vi "Handle Lask Ack.vi"(8 "error in (no error)":errorcluster, 10 "Last Ack":refnum<class "Last Ack.lvclass">, 11 "cRIO-CO2 in":refnum<class "cRIO-CO2.lvclass">) -> (0 "error out":errorcluster, 3 "cRIO-CO2 out":refnum<class "cRIO-CO2.lvclass">)   [LabVIEW 2015, in "cRIO-Carbondioxide.lvlib" / "cRIO-CO2.lvlib" / "cRIO-CO2.lvclass"]
uses:
  cRIO-CO2.lvclass
  <vilib>/ActorFramework/LastAck/Last Ack.lvclass
  CO2 Actor/CO2 Actor.lvclass
  <vilib>/ActorFramework/LastAck/Last Ack.lvclass/Last Ack.ctl
  CO2 Actor/CO2 Actor.lvclass/CO2 Actor.ctl
  cRIO-CO2.lvclass/cRIO-CO2.ctl
  <vilib>/ActorFramework/Message Enqueuer/Message Enqueuer.lvclass/Message Enqueuer.ctl
  <vilib>/ActorFramework/Message Enqueuer/Enqueue.vi
  <vilib>/ActorFramework/Message Priority Queue/Priority Enqueue.vi
  <vilib>/ActorFramework/Stop Msg/Stop Msg.lvclass
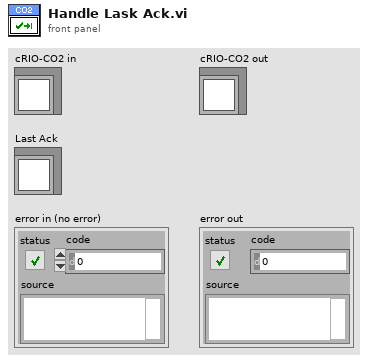
[diagram p1: front panel]
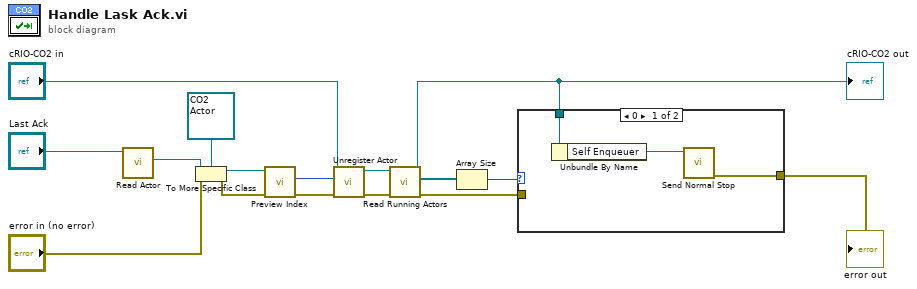
[diagram p0: block diagram]
diagram:
  n1 = call <vilib>:"Read Actor.vi"("Last Ack"="Last Ack") -> ("Actor"=w14:refnum<class "Actor.lvclass">)  [unwired: 10 in]
  n2 = To More Specific Class(target class=refnum<class "CO2 Actor.lvclass"> refnum ("CO2 Actor.lvclass"), reference=w14, error in="error in (no error)") -> (specific class reference=w12:refnum<class "CO2 Actor.lvclass">, error out=w13:errorcluster)
  n3 = call "Preview Index.vi"("error in (no error)"=w13, "CO2 Actor in"=w12) -> ("error out"=w11:errorcluster, "Index"=w9:i32)  [unwired: 7 in, 1 out]
  n4 = call "Unregister Actor.vi"("error in (no error)"=w11, "Index"=w9, "cRIO-CO2 in"="cRIO-CO2 in") -> ("error out"=w8:errorcluster, "cRIO-CO2 out"=w7:refnum<class "cRIO-CO2.lvclass">)  [unwired: 7 in]
  n5 = call "Read Running Actors.vi"("error in (no error)"=w8, "cRIO-CO2 in"=w7) -> ("error out"=w2:errorcluster, "Running Actors"=w6:refnum<class "CO2 Actor.lvclass">[], "cRIO-CO2 out"=w4:refnum<class "cRIO-CO2.lvclass">)  [unwired: 7 in]
  "cRIO-CO2 out" <- w4
  n6 = Array Size(array=w6) -> (size(s)=w5:i32)
  n7 = case shown="0" w5 {
    tunnel: w4 -> [w19 _]
    tunnel: [w17 _] -> w1
    tunnel: w2 -> [_ _]
    frame 0 {
      n8 = Unbundle By Name(w19) -> ("Self Enqueuer"=w18:refnum<class "Message Enqueuer.lvclass">)
      n9 = call <vilib>:"Send Normal Stop.vi"("Message Enqueuer"=w18) -> ("error out"=w17:errorcluster)  [unwired: 10 in]
    }
    frame 1, Default {
    }
  }
  "error out" <- w1
